vi "Spartan HTTP Config File.vi"() -> (1 "HTTP Configuration File":path)   [LabVIEW 2011]
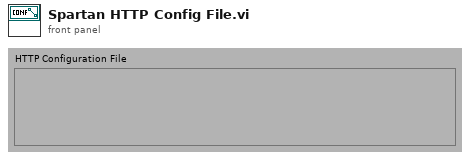
[diagram p1: front panel]
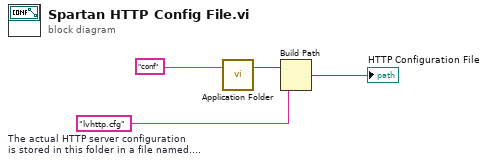
[diagram p0: block diagram]
diagram:
  w3 = "lvhttp.cfg"  # The actual HTTP server configuration is stored in this folder in a file named....
  n1 = call "Application Folder.vi"("Relative Path (\"\" - Folder)"="conf" ("name or relative path")) -> ("Application Folder"=w2:path)  [unwired: 2 in]
  n2 = Build Path(base path=w2, name or relative path=w3) -> (appended path=→"HTTP Configuration File":path)
